vi "InitialSensorCheck.vi"(4 "LinPot mm (center to finger) RIGHT":dbl, 5 "LinPot mm (center to finger) LEFT":dbl, 8 "Force bias PS_R":dbl, 9 "Force bias GR_R":dbl, 10 "Force bias PS_L":dbl, 11 "Force bias GR_L":dbl) -> (2 "Potentiometer Faulty":bool, 3 "Force Sensor Faulty":bool)   [LabVIEW 2019]
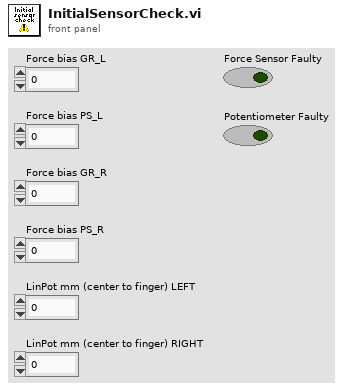
[diagram p1: front panel]
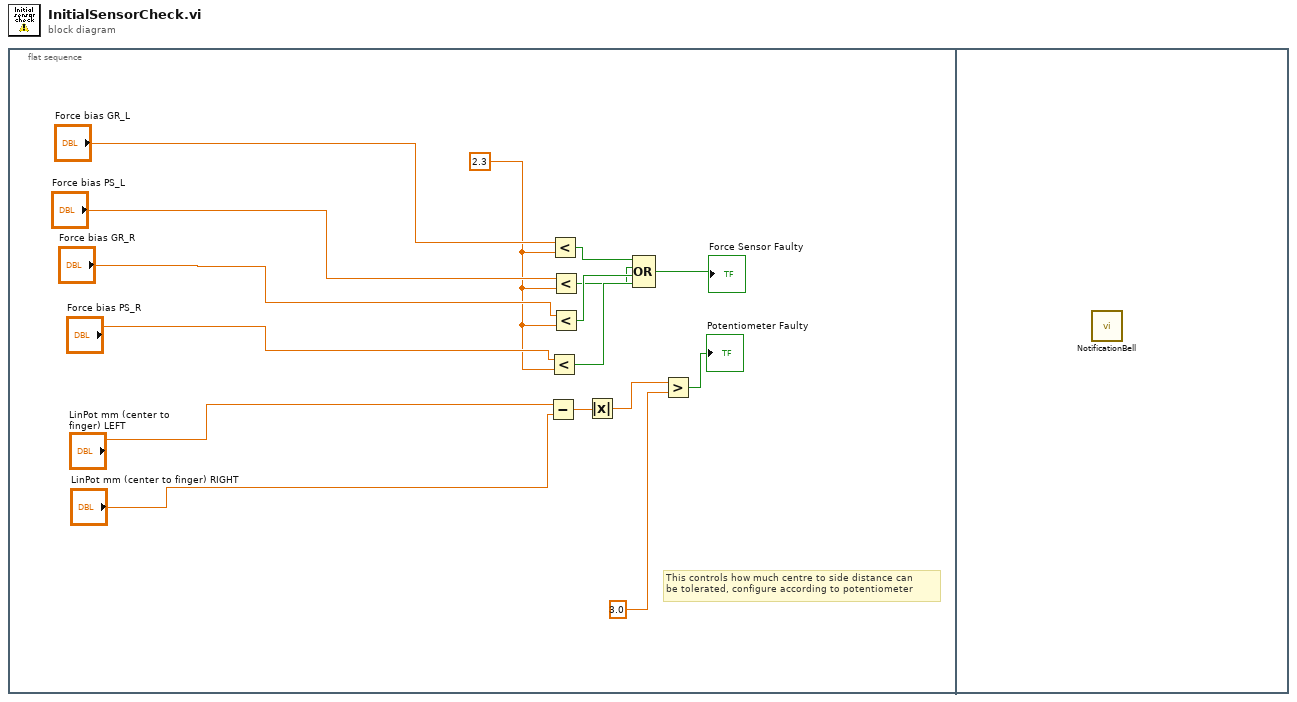
[diagram p0: block diagram]
diagram:
  n1 = flat-sequence {
    frame #0 {
      w1 = 2.3 ("y")
      # "This controls how much centre to side distance can \nbe tolerated, configure according to potentiometer"
      n2 = Subtract(x="LinPot mm (center to finger) LEFT", y="LinPot mm (center to finger) RIGHT") -> (x-y=w5:dbl)
      n3 = Less?(x="Force bias PS_R", y=w1) -> (x < y?=w9:bool)
      n4 = Less?(x="Force bias GR_L", y=w1) -> (x < y?=w6:bool)
      n5 = Less?(x="Force bias PS_L", y=w1) -> (x < y?=w7:bool)
      n6 = Less?(x="Force bias GR_R", y=w1) -> (x < y?=w8:bool)
      n7 = Absolute Value(x=w5) -> (abs(x)=w11:dbl)
      n8 = Compound Arithmetic op=OR(w6, w7, w8, w9) -> (→"Force Sensor Faulty":bool)
      n9 = Greater?(x=w11, y=3.0) -> (0:→"Potentiometer Faulty":bool)
    }
    frame #1 {
      n10 = call "NotificationBell.vi"() -> ()  [unwired: 12 in]
    }
  }
